vi "Find_Peak.vi"() -> ()   [LabVIEW 2010]
uses:
  <vilib>/Analysis/NI_AALPro.lvlib
panel:
  in  "Y array":dbl[](array[numeric]) format="%.2f"
  in  "X array":dbl[](array[numeric]) format="%.2f"
  out "XY Graph":cluster{dbl[], dbl[]}[](graph)
  out "Max Correlation":dbl format="%.2f"
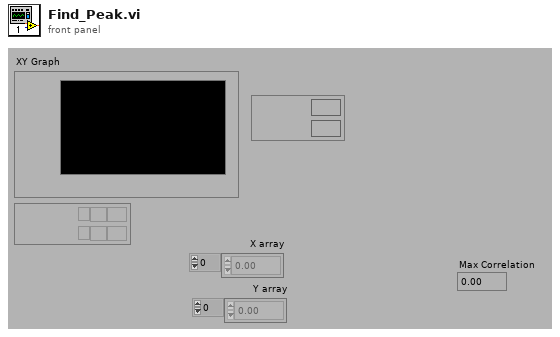
[diagram p1: front panel]
types:
  T1 = cluster{"X array":dbl[], "Best Polynomial Fit":dbl[]}
  T2 = cluster{"X array":dbl[], "Best Polynomial Fit":dbl[]}[]
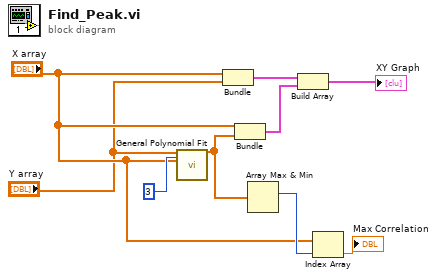
[diagram p0: block diagram]
diagram:
  n1 = call <vilib>:"General Polynomial Fit.vi"("Y"="Y array", "polynomial order"=3, "X"="X array") -> ("Best Polynomial Fit"=w7:dbl[])  [unwired: 9 in, 3 out]
  n2 = Bundle("X array"="X array", "Y array"="Y array") -> (w3:cluster{"X array":dbl[], "Y array":dbl[]})  [unwired: 1 in]
  n3 = Bundle("X array"="X array", "Best Polynomial Fit"=w7) -> (w5:T1)  [unwired: 1 in]
  n4 = Array Max & Min(array=w7) -> (max index (indices)=w8:i32)  [unwired: 3 out]
  n5 = Build Array(w3, w5) -> (→"XY Graph":T2)
  n6 = Index Array(array="X array", index=w8) -> (element=→"Max Correlation":dbl)
